vi "enable error reporting.vi"(8 "error in":errorcluster, 9 "tag":string, 10 "module ID":string, 11 "Standard Engine Configuration in":refnum<class "Standard Engine Configuration.lvclass">) -> (0 "error out":errorcluster, 3 "Standard Engine Configuration out":refnum<class "Standard Engine Configuration.lvclass">)   [LabVIEW 2013, in "Standard Engine Configuration.lvclass"]
uses:
  Standard Engine Configuration.lvclass
  <vilib>/NI/Tag Bus Module Framework/channel/channel classification.ctl
  <vilib>/NI/Tag Bus/tag/Data Type.ctl
  <vilib>/NI/Tag Bus/tag/tag descriptor.lvclass
  <vilib>/NI/Configuration Framework/serializable configuration/NISE_CEF_serializable configuration.lvclass/NISE_CEF_serializable configuration.ctl
  <vilib>/NI/Configuration Framework/serializable configuration/NISE_CEF_serializable configuration.lvclass
  Standard Engine Configuration.lvclass/Standard Engine Configuration.ctl
  <vilib>/NI/Module Execution Interface/Engine Configuration/engine configuration.lvclass
  <vilib>/NI/Tag Bus Module Framework/channel/TBM channel.lvclass
  <vilib>/NI/Configuration Framework/NISE_CEF_TreeControl.lvlib
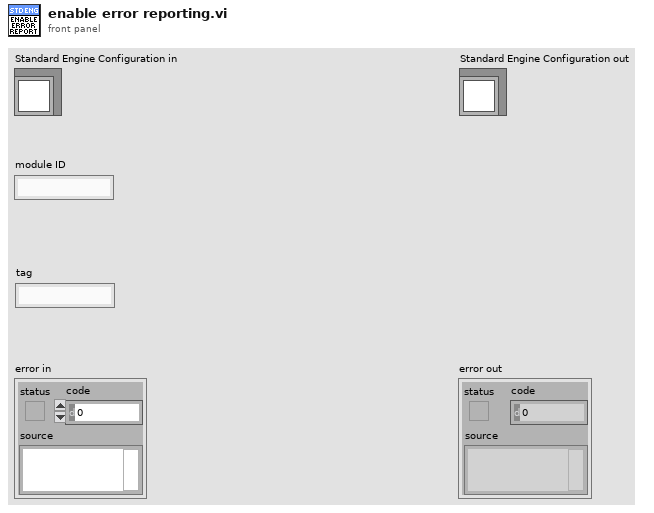
[diagram p1: front panel]
types:
  T1 = typedef "TBM channel.lvclass/channel classification.ctl" = enum16{"input data", "output data", "processing parameter", "processing result"}
  T2 = typedef "tag bus.lvlib/tag descriptor.lvclass/Data Type.ctl" = enum16{"Double", "Single", "I64", "I32", "I16", "I8", "U64", "U32", "U16", "U8", "Boolean", "String", "Array of Double", "Array of Single", "Array of I64", "Array of I32", "Array of I16", "Array of I8", "Array of U64", "Array of U32", "Array of U16", "Array of U8", "Array of Boolean", "Array of String"}
  T3 = typedef "Standard Engine Configuration.lvclass/Module Specific Configuration.ctl" = cluster{"Module ID":string, "Module Decimation":T4, "Module Error Configuration":T5, "execution order priority":i32, "async?":bool, "error tag":string}
  T4 = typedef "Standard Engine Configuration.lvclass/Module Decimation.ctl" = cluster{"Decimation":u16, "Offset":u16}
  T5 = typedef "Standard Engine Configuration.lvclass/Module Error Configuration.ctl" = cluster{"Module Error Configuration":T6[]}
  T6 = typedef "Standard Engine Configuration.lvclass/Error Actions By Category.ctl" = cluster{"error classification":T7, "Error Actions":T8[]}
  T7 = typedef "TBM module execution interface.lvclass/error classification.ctl" = enum16{"unknown", "none", "trivial", "recoverable", "critical"}
  T8 = typedef "Standard Engine Configuration.lvclass/Error Actions.ctl" = enum16{"Clear", "Notify", "Stop Component", "Stop Engine", "Safe State", "Attempt Recovery"}
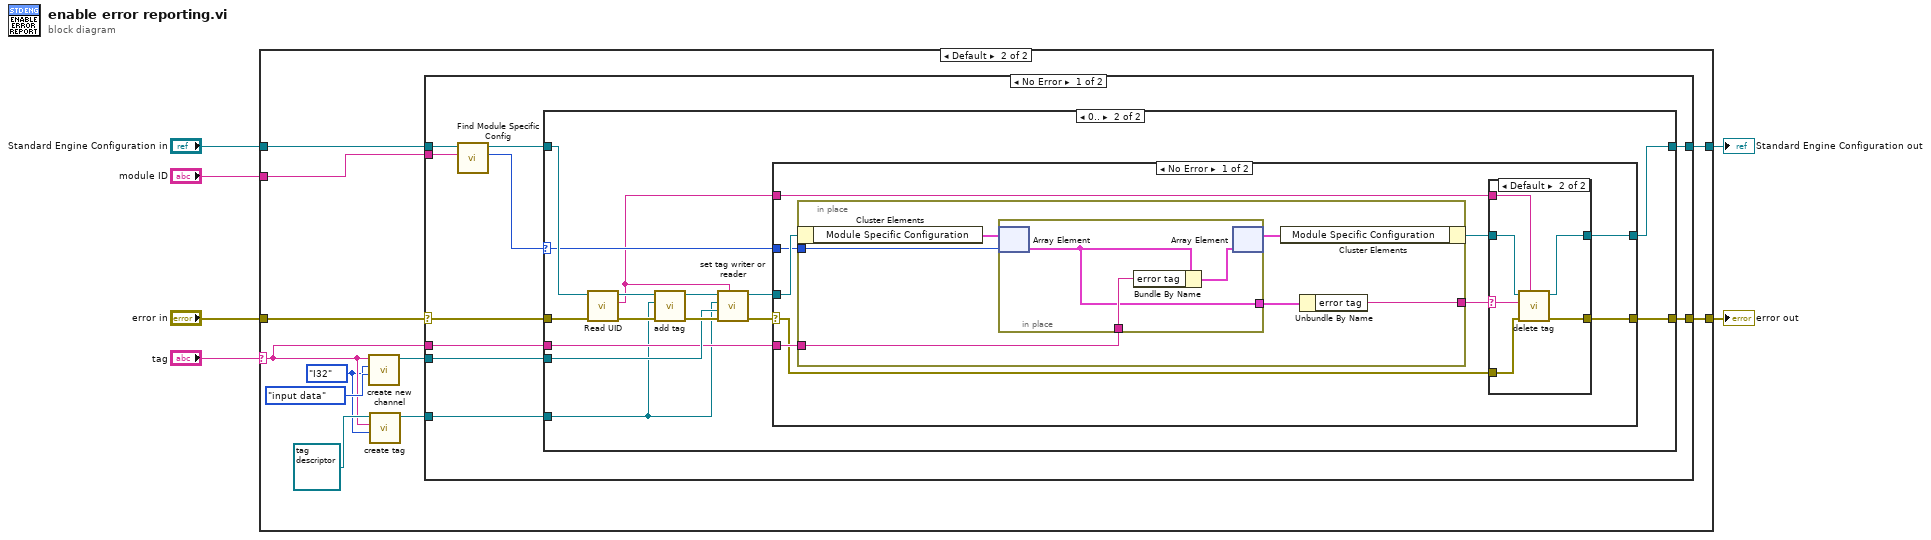
[diagram p0: block diagram]
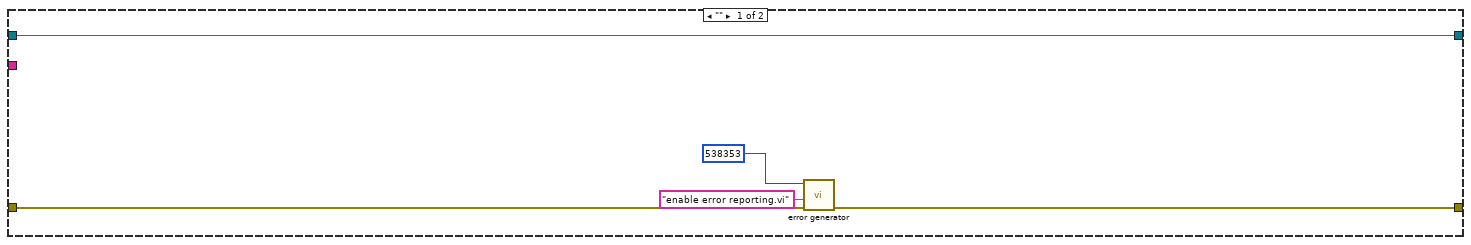
[diagram p2: hidden frame]
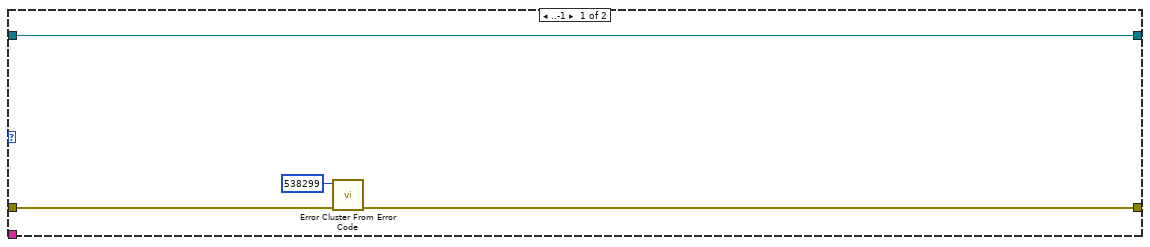
[diagram p3: hidden frame]
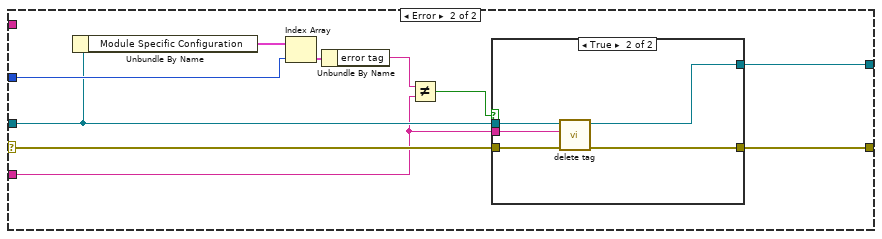
[diagram p5: hidden frame]
diagram:
  n1 = case shown="Default" "tag" {
    selector: "tag" -> [_ w14]
    tunnel: "Standard Engine Configuration in" -> [w11 w22]
    tunnel: "module ID" -> [_ w21]
    tunnel: "error in" -> [w10 w20]
    tunnel: [w11 w19] -> w3
    tunnel: [w9 w18] -> w2
    frame "" {
      n2 = call <vilib>:"error generator.vi"("error in"=w10, "source"="enable error reporting.vi", "error code (0)"=538353) -> ("error out"=w9:errorcluster)  [unwired: 6 in]
    }
    frame Default {
      w12 = Data_Type."I32" ("data type")
      n3 = call <vilib>:"create new channel.vi"("channel classification"=channel_classification."input data", "data type"=w12, "channel name"=w14) -> ("channel"=w17:refnum<class "TBM channel.lvclass">)  [unwired: 8 in]
      n4 = call-dynamic "create tag.vi"("data type"=w12, "name"=w14, "tag descriptor in"=refnum<class "tag descriptor.lvclass"> refnum) -> ("tag descriptor out"=w13:refnum<class "tag descriptor.lvclass">)  [unwired: 7 in, 1 out]
      n5 = case shown="No Error" w20 {
        selector: w20 -> [w28 w96]
        tunnel: w22 -> [w32 w95]
        tunnel: w21 -> [w31 _]
        tunnel: [w26 w95] -> w19
        tunnel: [w27 w96] -> w18
        tunnel: w17 -> [w25 _]
        tunnel: w14 -> [w24 _]
        tunnel: w13 -> [w23 _]
        frame No Error {
          n6 = call "Find Module Specific Config.vi"("Module ID"=w31, "Standard Engine Repo Data in"=w32) -> ("Index"=w29:i32, "Standard Engine Repo Data out"=w30:refnum<class "Standard Engine Configuration.lvclass">)  [unwired: 8 in]
          n7 = case shown="0.." w29 {
            selector: w29 -> [_ w41]
            tunnel: w30 -> [w36 w47]
            tunnel: w28 -> [w35 w51]
            tunnel: [w34 w42] -> w27
            tunnel: [w36 w43] -> w26
            tunnel: w25 -> [_ w40]
            tunnel: w24 -> [_ w39]
            tunnel: w23 -> [_ w37]
            frame ..-1 {
              n8 = call <vilib>:"Error Cluster From Error Code.vi"("error in (no error)"=w35, "error code (0)"=538299) -> ("error out"=w34:errorcluster)  [unwired: 7 in]
            }
            frame 0.. {
              n9 = call <vilib>:"Read UID.vi"("error in"=w51, "configuration in"=w47) -> ("error out"=w48:errorcluster, "instance id"=w38:string, "configuration out"=w46:refnum<class "Standard Engine Configuration.lvclass">)  [unwired: 7 in]
              n10 = call <vilib>:"add tag.vi"("error in"=w48, "tag descriptor"=w37, "engine configuration in"=w46) -> ("error out"=w50:errorcluster, "engine configuration out"=w49:refnum<class "Standard Engine Configuration.lvclass">)  [unwired: 7 in]
              n11 = call <vilib>:"set tag writer or reader.vi"("module GUID"=w38, "error in"=w50, "channel"=w40, "tag descriptor"=w37, "engine configuration in"=w49) -> ("error out"=w45:errorcluster, "engine configuration out"=w44:refnum<class "Standard Engine Configuration.lvclass">)  [unwired: 5 in]
              n12 = case shown="No Error" w45 {
                selector: w45 -> [w54 w82]
                tunnel: w44 -> [w60 w83]
                tunnel: [w56 w80] -> w43
                tunnel: [w55 w81] -> w42
                tunnel: w41 -> [w59 w86]
                tunnel: w39 -> [w58 w79]
                tunnel: w38 -> [w53 _]
                frame No Error {
                  n13 = in-place {
                    in-place-border: w59 -> [w72]
                    in-place-border: w58 -> [w71]
                    in-place-border: [w69] -> w52
                    n14 = in-place-cluster #1(w60) -> ("Module Specific Configuration"=w74:T3[])
                    n15 = in-place {
                      in-place-border: w71 -> [w76]
                      in-place-border: [w75] -> w70
                      n16 = in-place-array #2(w74, w72) -> (w75:T3)
                      n17 = Bundle By Name(cluster=w75, "error tag"=w76) -> (w77:T3)
                      n18 = in-place-array #2(w77) -> (w73:T3[])  [unwired: 1 out]
                    }
                    n19 = in-place-cluster #1("Module Specific Configuration"=w73) -> (w57:refnum<class "Standard Engine Configuration.lvclass">)
                    n20 = Unbundle By Name(w70) -> ("error tag"=w69:string)
                  }
                  n21 = case shown="Default" w52 {
                    selector: w52 -> [_ w63]
                    tunnel: w57 -> [w62 w68]
                    tunnel: [w62 w67] -> w56
                    tunnel: [w61 w66] -> w55
                    tunnel: w54 -> [w61 w65]
                    tunnel: w53 -> [_ w64]
                    frame "" {
                    }
                    frame Default {
                      n22 = call <vilib>:"delete tag.vi"("owner ID"=w64, "error in"=w65, "tag name"=w63, "engine configuration in"=w68) -> ("error out"=w66:errorcluster, "engine configuration out"=w67:refnum<class "Standard Engine Configuration.lvclass">)  [unwired: 6 in]
                    }
                  }
                }
                frame Error {
                  n23 = Unbundle By Name(w83) -> ("Module Specific Configuration"=w87:T3[])
                  n24 = Index Array(array=w87, index=w86) -> (element=w85:T3)
                  n25 = Unbundle By Name(w85) -> ("error tag"=w84:string)
                  n26 = Not Equal?(x=w84, y=w79) -> (x != y?=w78:bool)
                  n27 = case shown="True" w78 {
                    tunnel: w83 -> [w89 w94]
                    tunnel: w82 -> [w88 w93]
                    tunnel: [w88 w92] -> w81
                    tunnel: [w89 w91] -> w80
                    tunnel: w79 -> [_ w90]
                    frame False {
                    }
                    frame True {
                      n28 = call <vilib>:"delete tag.vi"("error in"=w93, "tag name"=w90, "engine configuration in"=w94) -> ("error out"=w92:errorcluster, "engine configuration out"=w91:refnum<class "Standard Engine Configuration.lvclass">)  [unwired: 7 in]
                    }
                  }
                }
              }
            }
          }
        }
        frame Error {
        }
      }
    }
  }
  "error out" <- w2
  "Standard Engine Configuration out" <- w3
